vi "Read Child Attributes Map.vi"(11 "Base Actor in":refnum<class "Base Actor.lvclass">) -> (2 "Child Attributes Map":T1)   [LabVIEW 2020, in "jettl.lvlib" / "Base jettl Actor.lvlib" / "Base Actor.lvlib" / "Base Actor.lvclass"]
uses:
  Base Actor.lvclass
  Base Actor.lvclass/Base Actor.ctl
  Msg/Msg.lvclass
  Transport/Transport.lvclass
  Actor/Actor.lvclass
  Child Actor Attributes Map.ctl
  jettl.lvlib
  Actor Attributes.ctl
  Msgs.ctl
  Msg Names.ctl
  Unified Layer.ctl
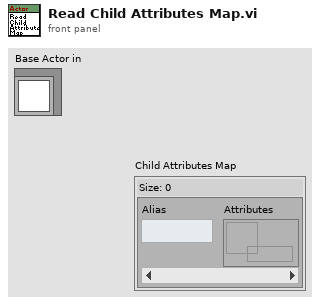
[diagram p1: front panel]
types:
  T1 = typedef "jettl.lvlib/Child Actor Attributes Map.ctl" = map{string, refnum<data-value>}
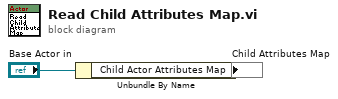
[diagram p0: block diagram]
diagram:
  n1 = Unbundle By Name("Base Actor in") -> ("Child Actor Attributes Map"=→"Child Attributes Map":refnum<data-value>)
